vi "Destroy User Events.vi"(11 "UI Template in":refnum<class "UI_Waveform.lvclass">) -> (3 "UI Template out":refnum<class "UI_Waveform.lvclass">)   [LabVIEW 2021, in "UI_Waveform.lvclass"]
uses:
  UI_Waveform.lvclass
  UI_Waveform.lvclass/UI_Waveform.ctl
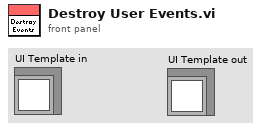
[diagram p1: front panel]
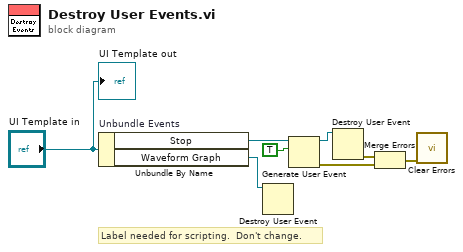
[diagram p0: block diagram]
diagram:
  # "Label needed for scripting.  Don't change."
  n1 = Unbundle By Name "Unbundle Events"("UI Template in") -> ("Stop"=w6:refnum<user-event>, "Waveform Graph"=w1:refnum<user-event>)
  n2 = Destroy User Event(user event=w1) -> ()  [unwired: 1 in, 1 out]
  n3 = Generate User Event(user event=w6, event data cluster=TRUE ("event data")) -> (user event out=w7:refnum<user-event>, error out=w2:errorcluster)  [unwired: 2 in]
  n4 = Destroy User Event(user event=w7) -> (error out=w4:errorcluster)  [unwired: 1 in]
  n5 = Merge Errors(w4, w2) -> (w3:errorcluster)
  n6 = call <vilib>:"Clear Errors.vi"("error in (no error)"=w3) -> ()  [unwired: 5 in, 2 out]
  "UI Template out" <- "UI Template in"
